vi "Init.vi"(10 "Input":refnum<data-value>) -> (3 "TEMPLATE Msg Input":refnum<class "TEMPLATE Msg Input.lvclass">)   [LabVIEW 2020, in "_Template.lvlib" / "Templates.lvlib" / "TEMPLATE jettl Msg.lvlib" / "TEMPLATE Msg Input.lvclass"]
uses:
  TEMPLATE Msg Input.lvclass
  TEMPLATE Msg Input.lvclass/TEMPLATE Msg Input.ctl
  Input.ctl
  TEMPLATE jettl Msg.lvlib
panel:
  # "This front panel should not be manipulated."
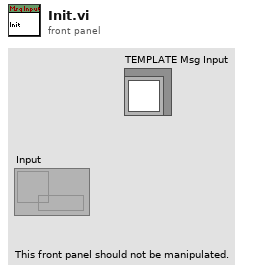
[diagram p1: front panel]
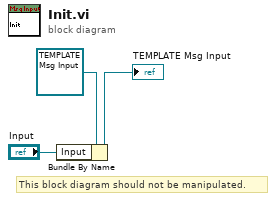
[diagram p0: block diagram]
diagram:
  # "This block diagram should not be manipulated."
  n1 = Bundle By Name(cluster=refnum<class "TEMPLATE Msg Input.lvclass"> refnum ("TEMPLATE Msg Input"), "Input"="Input") -> (→"TEMPLATE Msg Input":refnum<class "TEMPLATE Msg Input.lvclass">)
